vi "Actor Core.vi"(8 "error in":errorcluster, 11 "Kasli Wrapper in":refnum<class "Kasli Wrapper 2.0.lvclass">) -> (0 "error out":errorcluster, 3 "Actor out":refnum<class "Actor.lvclass">)   [LabVIEW 2020, in "TALOS.lvlib" / "Kasli Wrapper 2.0.lvlib" / "Kasli Wrapper 2.0.lvclass"]
doc: "(<B>Filename</B>: Actor Framework.lvlib:Actor.lvclass:Actor Core.vi)\n\nReceives messages to the actor, reacts to them, and initiates any error handling that may shut the actor down.\n\nDescendant classes may override this VI to append parallel tasks for the actor to complete while it handles messages. Overrides use the Call Parent Class Method node."
uses:
  Kasli Wrapper 2.0.lvclass
  C:/LabVIEW Code/TALOS/talos/Father of all uServices/Father of all uServices/Father of all uServices.lvclass
  C:/LabVIEW Code/TALOS/builds/Actor Framework PPL/Actor Framework.lvlibp/1abvi3w/vi.lib/ActorFramework/Actor/Actor.lvclass
  builds/Actor Framework PPL/Actor Framework.lvlibp/1abvi3w/vi.lib/ActorFramework/Actor/Actor.lvclass
  Kasli Wrapper 2.0.lvclass/Kasli Wrapper 2.0.ctl
  Kasli Wrapper 2.0 Consumer Case Selector.ctl
  Father of all uServices/Father of all uServices Messages/Consumer Msg/Consumer Msg.lvclass/Consumer Msg.ctl
  Ancestor/Ancestor/Ancestor.lvclass/Ancestor.ctl
  builds/Actor Framework PPL/Actor Framework.lvlibp/1abvi3w/vi.lib/ActorFramework/Message Enqueuer/Message Priority.ctl
  Ancestor/Ancestor Messages/Process EH Error Msg/Process EH Error Msg.lvclass/Process EH Error Msg.ctl
  Father of all uServices/Father of all uServices Messages/Consumer Msg/Send Consumer.vi
  Support VIs/Generate Error.vi
  FGV/Error Memory/Get Error Description.vi
  Support VIs/Get PC name.vi
  Ancestor/Ancestor/Read ID.vi
  Support VIs/Get Class Name.vi
  <vilib>/Utility/error.llb/Clear Errors.vi
  FGV/Error Memory/Error Memory Core.vi
  <vilib>/AdvancedString/Delimited String to 1D String Array.vi
  Support VIs/Circus Root Path.vi
  FGV/Error Memory/Error Crt Lvl checker.vi
  FGV/Error Memory/Error Memory Core.vi/40c8088d-b597-4017-91af-faa98e00292e.vi
  FGV/Error Memory/Error Memory Core.vi/d4a3ab98-063c-4e44-b43d-fbdcfe6c2be2.vi
  Father of all uServices/Father of all uServices/Father of all uServices.lvclass
  <userlib>/_OpenG.lib/lvdata/lvdata.llb/Get Strings from Enum__ogtk.vi
  builds/Actor Framework PPL/Actor Framework.lvlibp/1abvi3w/vi.lib/ActorFramework/Message Enqueuer/Enqueue.vi
  Support VIs/Global Memory.vi
  <vilib>/Utility/LVClass/Get LV Class Name.vi
  Support VIs/Is in Packed Library.vi
  Support VIs/TALOS Root path.vi
  Support VIs/Read CSV worksheet.vi
  Support VIs/Global Constants.vi
  <vilib>/Utility/error.llb/General Error Handler.vi
  Support VIs/Error Log.vi
  Father of all uServices/Father of all uServices Messages/Consumer Msg/Consumer Msg.lvclass
  Ancestor/Ancestor/Ancestor.lvclass
  <vilib>/Comparison/Equal/Equal Functor/Equal Functor.lvclass
  Ancestor/Ancestor Messages/Process EH Error Msg/Process EH Error Msg.lvclass
  TALOS.lvlib
  builds/Actor Framework PPL/Actor Framework.lvlibp/1abvi3w/vi.lib/ActorFramework/Message Enqueuer/Message Enqueuer.lvclass
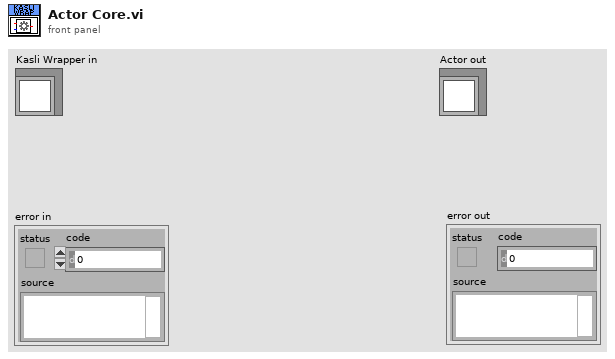
[diagram p1: front panel]
types:
  T1 = cluster{"Stop Kasli Wrapper EH user event":refnum<user-event>, "Resubscribe Kasli Public Events user event":refnum<user-event>, "Kasli public events":cluster{"stdout event":refnum<user-event>, "stderr event":refnum<user-event>, "process_exit event":refnum<user-event>}}
  T2 = typedef "TALOS.lvlib/Kasli Wrapper 2.0.lvlib/Kasli Wrapper 2.0.lvclass/Kasli Wrapper 2.0 Consumer Case Selector.ctl" = enum16{"Init", "Submit Script", "Restart Master", "Master StdOut", "Master StdErr", "Client StdOut", "Client StdErr", "Start Logging", "Stop Logging", "Terminate Script", "Close", "Master ProcessExit"}
  T3 = typedef "Actor Framework.lvlibp/Message Enqueuer.lvclass/Message Priority.ctl" = enum16{"Low", "Normal", "High"}
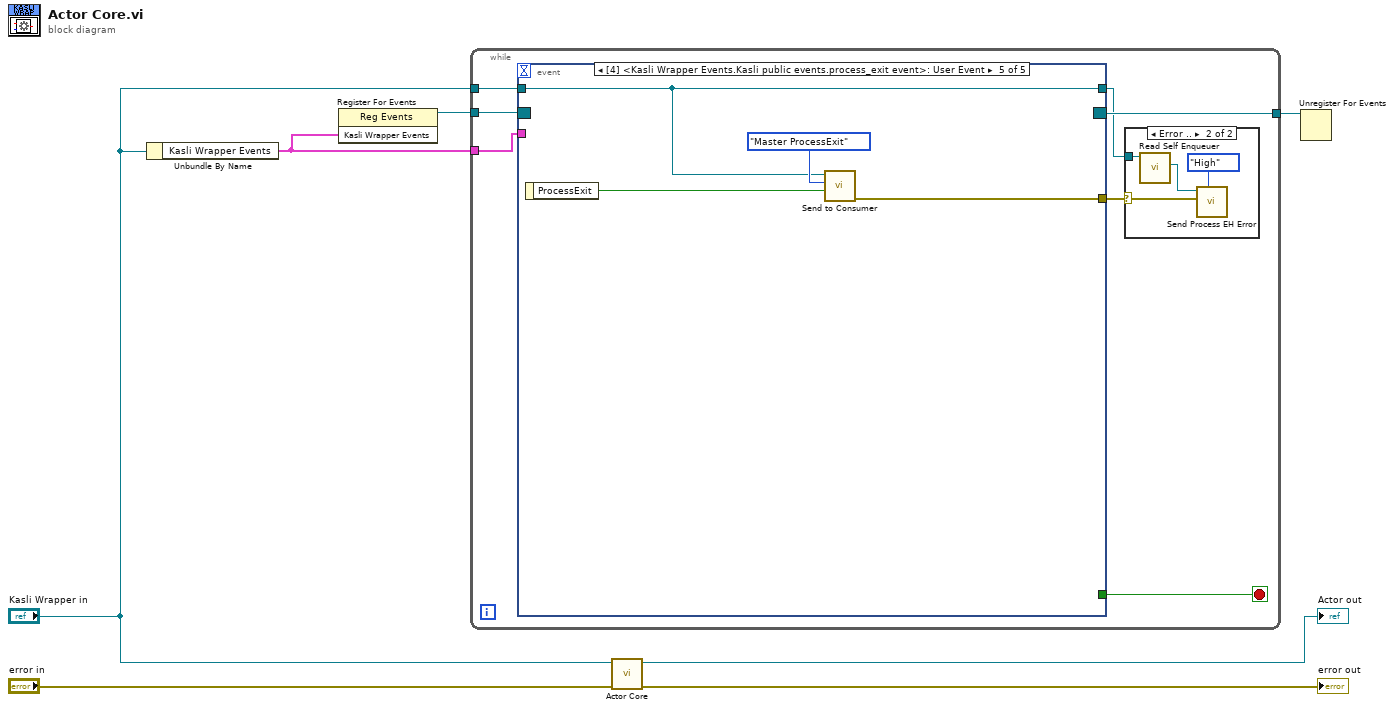
[diagram p0: block diagram]
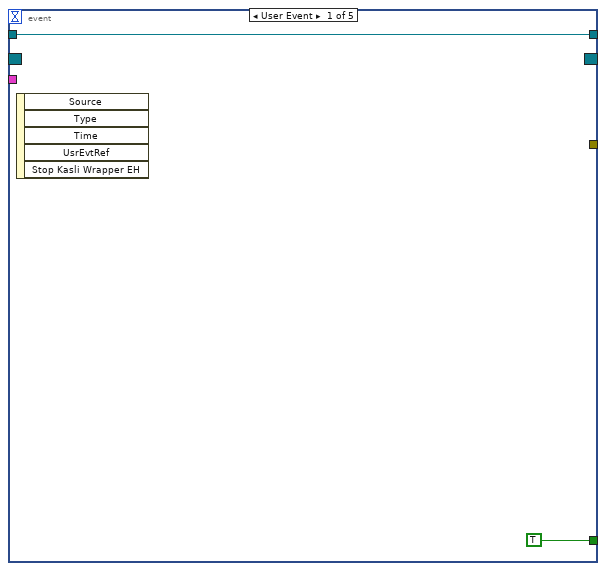
[diagram p2: hidden frame]
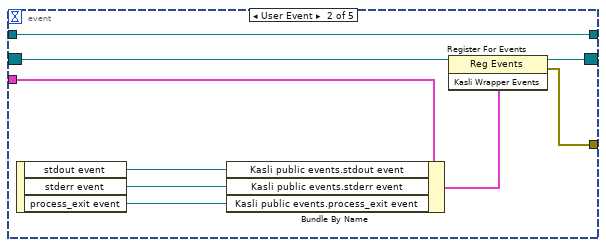
[diagram p3: hidden frame]
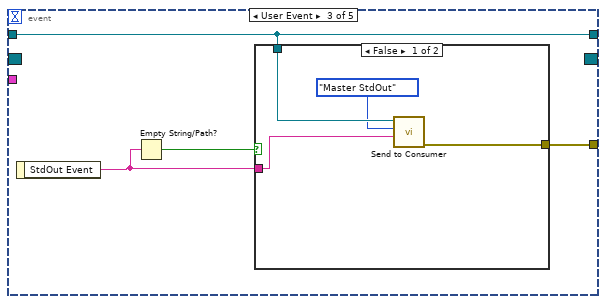
[diagram p4: hidden frame]
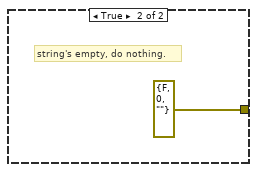
[diagram p5: hidden frame]
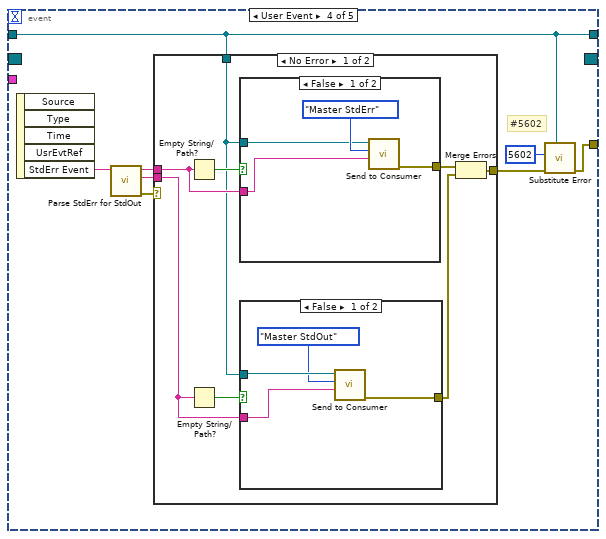
[diagram p6: hidden frame]
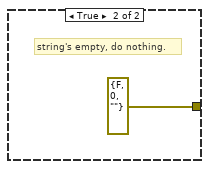
[diagram p7: hidden frame]
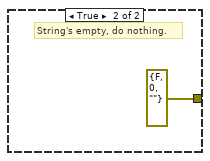
[diagram p8: hidden frame]
diagram:
  n1 = Unbundle By Name("Kasli Wrapper in") -> ("Kasli Wrapper Events"=w4:T1)
  n2 = register-events(w4) -> (reference out=w5:refnum<event-registration>)  [unwired: 2 in, 1 out]
  n3 = while {
    tunnel: w5 -> [w14]
    tunnel: w4 -> [w12]
    tunnel: [w11] -> w3
    tunnel: "Kasli Wrapper in" -> [w10]
    stop <- w13 stop-if-true
    n4 = event shown="[4] <Kasli Wrapper Events.Kasli public events.process_exit event>: User Event" {
      selector: w14 -> [_ w25 _ _ _]
      dyn-events: [_ w24 _ _ _] -> w11
      timeout: _ -> [_ _ _ _ _]
      tunnel: [TRUE _ _ _ _] -> w13
      tunnel: w12 -> [_ w23 _ _ _]
      tunnel: [_ w18 w29 w37 w62] -> w8
      tunnel: w10 -> [w15 w17 w26 w36 w63]
      tunnel: [w15 w17 w26 w36 w63] -> w9
      event User Event {
        n5 = event-data() -> ()  [unwired: 1 in, 5 out]
      }
      event User Event {
        n6 = event-data() -> ("stdout event"=w22:refnum<user-event>, "stderr event"=w21:refnum<user-event>, "process_exit event"=w20:refnum<user-event>)  [unwired: 1 in]
        n7 = Bundle By Name(cluster=w23, "Kasli public events.stdout event"=w22, "Kasli public events.stderr event"=w21, "Kasli public events.process_exit event"=w20) -> (w19:T1)
        n8 = register-events(reference=w25, w19) -> (reference out=w24:refnum<event-registration>, error out=w18:errorcluster)  [unwired: 1 in]
      }
      event User Event {
        n9 = event-data() -> ("StdOut Event"=w27:string)  [unwired: 1 in]
        n10 = Empty String/Path?(string/path=w27) -> (empty?=w28:bool)
        n11 = case shown="False" w28 {
          tunnel: [w31 errorcluster {"status"=FALSE, "code"=0, "source"=""} ("error IO")] -> w29
          tunnel: w27 -> [w30 _]
          tunnel: w26 -> [w33 _]
          frame False {
            n12 = call "Send to Consumer.vi"("Data"=w30, "Case ID"=Kasli_Wrapper_2.0_Consumer_Case_Selector."Master StdOut" ("Consumer Case Selector"), "uService Template in"=w33) -> ("error out"=w31:errorcluster)  [unwired: 7 in, 1 out]
          }
          frame True {
            # "string's empty, do nothing."
          }
        }
      }
      event User Event {
        # "#5602"
        n13 = event-data() -> ("StdErr Event"=w40:string)  [unwired: 1 in, 4 out]
        n14 = call "Parse StdErr for StdOut.vi"("StdErr Event"=w40) -> ("error out"=w39:errorcluster, "StdOut"=w42:string, "StdErr"=w41:string)  [unwired: 8 in]
        n15 = case shown="No Error" w39 {
          selector: w39 -> [_ w61]
          tunnel: w42 -> [w47 _]
          tunnel: w41 -> [w46 _]
          tunnel: w36 -> [w45 _]
          tunnel: [w44 w61] -> w38
          frame No Error {
            n16 = Empty String/Path?(string/path=w46) -> (empty?=w49:bool)
            n17 = Empty String/Path?(string/path=w47) -> (empty?=w48:bool)
            n18 = case shown="False" w49 {
              tunnel: w46 -> [w56 _]
              tunnel: w45 -> [w58 _]
              tunnel: [w57 errorcluster {"status"=FALSE, "code"=0, "source"=""} ("error out")] -> w50
              frame False {
                n19 = call "Send to Consumer.vi"("Data"=w56, "Case ID"=Kasli_Wrapper_2.0_Consumer_Case_Selector."Master StdErr" ("Consumer Case Selector"), "uService Template in"=w58) -> ("error out"=w57:errorcluster)  [unwired: 7 in, 1 out]
              }
              frame True {
                # "String's empty, do nothing."
              }
            }
            n20 = case shown="False" w48 {
              tunnel: [w51 errorcluster {"status"=FALSE, "code"=0, "source"=""} ("error IO")] -> w43
              tunnel: w47 -> [w52 _]
              tunnel: w45 -> [w54 _]
              frame False {
                n21 = call "Send to Consumer.vi"("Data"=w52, "Case ID"=Kasli_Wrapper_2.0_Consumer_Case_Selector."Master StdOut" ("Consumer Case Selector"), "uService Template in"=w54) -> ("error out"=w51:errorcluster)  [unwired: 7 in, 1 out]
              }
              frame True {
                # "string's empty, do nothing."
              }
            }
            n22 = Merge Errors(w50, w43) -> (w44:errorcluster)
          }
          frame Error {
          }
        }
        n23 = call "Substitute Error.vi"("LabVIEW Object"=w36, "error in (no error)"=w38, "Error Code"=5602) -> ("error out"=w37:errorcluster)  [unwired: 8 in]
      }
      event User Event {
        n24 = event-data() -> ("ProcessExit"=w64:bool)  [unwired: 1 in]
        n25 = call "Send to Consumer.vi"("Data"=w64, "Case ID"=Kasli_Wrapper_2.0_Consumer_Case_Selector."Master ProcessExit" ("Consumer Case Selector"), "uService Template in"=w63) -> ("error out"=w62:errorcluster)  [unwired: 7 in, 1 out]
      }
    }
    n26 = case shown="Error .." w8 {
      selector: w8 -> [_ w69]
      tunnel: w9 -> [_ w68]
      frame No Error {
      }
      frame Error {
        n27 = call "Read Self Enqueuer.vi"("Actor"=w68) -> ("Self Enqueuer"=w67:refnum<class "Message Enqueuer.lvclass">)  [unwired: 10 in]
        n28 = call "Send Process EH Error.vi"("Message Priority (Normal)"=Message_Priority."High", "Error to process"=w69, "Message Enqueuer"=w67) -> ()  [unwired: 7 in, 2 out]
      }
    }
  }
  n29 = call-parent "Actor Core.vi"("error in"="error in", "uService Template in"="Kasli Wrapper in") -> ("error out"=→"error out":errorcluster, "Actor out"=→"Actor out":refnum<class "Actor.lvclass">)  [unwired: 8 in]
  n30 = Unregister For Events(event registration refnum=w3) -> ()  [unwired: 1 in, 1 out]
